vi "Remove IDs from Data.vi"(3 "Data In":string[][](array[string])) -> (1 "Data Out":string[][](array[string]))   [LabVIEW 2013]
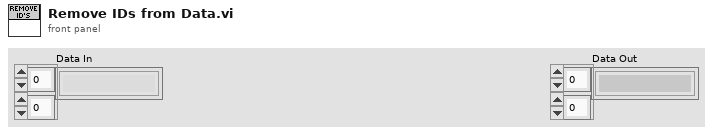
[diagram p1: front panel]
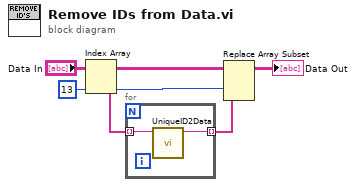
[diagram p0: block diagram]
diagram:
  w4 = 13 ("disabled index (col)")
  n1 = Index Array(array="Data In", index (col)=w4) -> (element=w3:string[])  [unwired: 1 in]
  n2 = for {
    tunnel: w3 -> [w7] mode=indexing
    tunnel: [w6] -> w2 mode=indexing
    n3 = call "UniqueID2Data.vi"("UniqueID"=w7) -> ("Data"=w6:string)  [unwired: 10 in]
  }
  n4 = Replace Array Subset(array="Data In", new element=w2, index (col)=w4) -> (→"Data Out":string[][])  [unwired: 1 in]
